vi "EminemExecute.vi"(8 "error in (no error)":errorcluster) -> (0 "error out":errorcluster)   [LabVIEW 2023]
panel:
  # "Click here to set min"
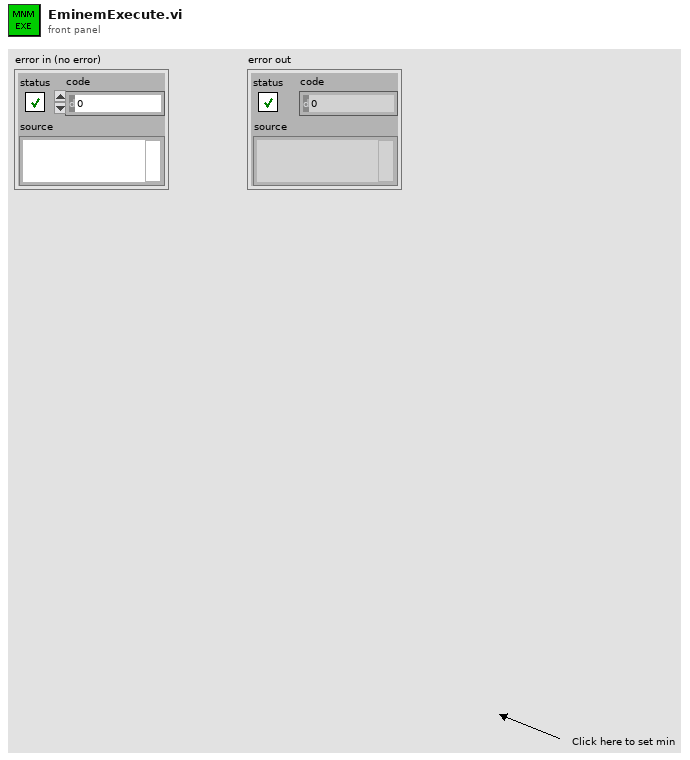
[diagram p1: front panel]
types:
  T1 = typedef "WPI_MotorControlDeviceRef.ctl" = cluster{"DeviceStatus":errorcluster, "Type":T2, "PWM":cluster{"PWM Channel":T3, "DeadBand":T4}, "CAN":cluster{"Device Number":u8, "SetOutput VI Ref":variant, "GetOutput VI Ref":variant, "Enable VI Ref":variant, "Disable VI Ref":variant, "Data":variant}, "Invert":bool, "DIO PWM":cluster{"PWM \"Enable\" Channel":T3, "DIOChannel":T5, "PWM Rate":dbl}}
  T2 = typedef "WPI_MotorControlType.ctl" = enum16{"PWM", "CAN", "DIO PWM"}
  T3 = typedef "FPGA_DIOPWMChannel.ctl" = enum8{"PWM 0", "PWM 1", "PWM 2", "PWM 3", "PWM 4", "PWM 5", "PWM 6", "PWM 7", "PWM 8", "PWM 9", "PWM MXP 0", "PWM MXP 1", "PWM MXP 2", "PWM MXP 3", "PWM MXP 4", "PWM MXP 5", "PWM MXP 6", "PWM MXP 7", "PWM MXP 8", "PWM MXP 9", "Invalid"}
  T4 = typedef "WPI_PWMDeadband.ctl" = cluster{"Name":string, "maxPositivePwm":i32, "minPositivePwm":i32, "centerPwm":i32, "maxNegativePwm":i32, "minNegativePwm":i32, "angularRange":u16}
  T5 = typedef "FPGA_DIOChannel.ctl" = enum8{"DIO 0", "DIO 1", "DIO 2", "DIO 3", "DIO 4", "DIO 5", "DIO 6", "DIO 7", "DIO 8", "DIO 9", "DIO MXP 0", "DIO MXP 1", "DIO MXP 2", "DIO MXP 3", "DIO MXP 4", "DIO MXP 5", "DIO MXP 6", "DIO MXP 7", "DIO MXP 8", "DIO MXP 9", "DIO MXP 10", "DIO MXP 11", "DIO MXP 12", "DIO MXP 13", "DIO MXP 14", "DIO MXP 15", "SPI Port CS1", "SPI Port CS2", "SPI Port CS3", "SPI Port MISO", "SPI Port MOSI", "Invalid"}
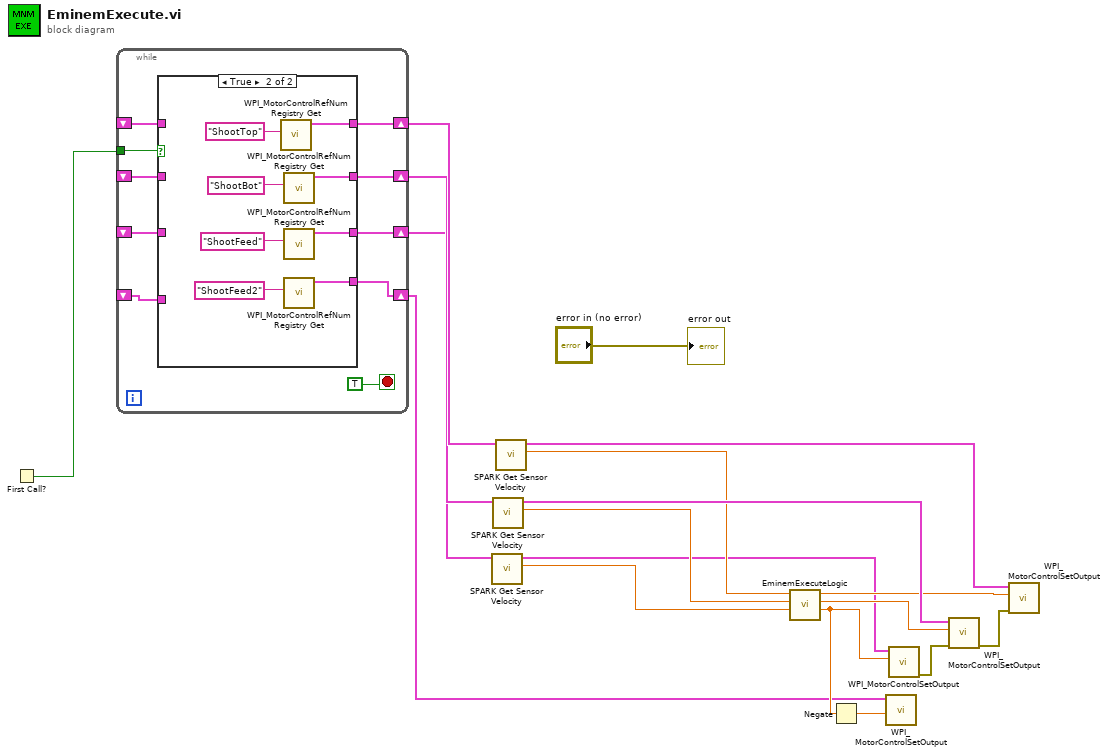
[diagram p0: block diagram]
diagram:
  n1 = First Call?() -> (First Call?: T/F=w14:bool)
  n2 = while {
    tunnel: w14 -> [w26]
    shift-right: [w28] -> w18
    shift-left: _ -> [w24]
    shift-right: [w27] -> w17
    shift-left: _ -> [w23]
    shift-right: [w22] -> w6
    shift-left: _ -> [w21]
    shift-right: [w20] -> w1
    shift-left: _ -> [w19]
    stop <- TRUE stop-if-true
    n3 = case shown="True" w26 {
      tunnel: [w32 w38] -> w28
      tunnel: [w31 w37] -> w27
      tunnel: w24 -> [w32 _]
      tunnel: w23 -> [w31 _]
      tunnel: [w30 w35] -> w22
      tunnel: w21 -> [w30 _]
      tunnel: [w29 w33] -> w20
      tunnel: w19 -> [w29 _]
      frame False {
      }
      frame True {
        n4 = call <vilib>:"WPI_MotorControlRefNum Registry Get.vi"("refnum name"="ShootTop") -> ("MotorControlDevRef"=w38:T1)  [unwired: 9 in, 1 out]
        n5 = call <vilib>:"WPI_MotorControlRefNum Registry Get.vi"("refnum name"="ShootBot") -> ("MotorControlDevRef"=w37:T1)  [unwired: 9 in, 1 out]
        n6 = call <vilib>:"WPI_MotorControlRefNum Registry Get.vi"("refnum name"="ShootFeed") -> ("MotorControlDevRef"=w35:T1)  [unwired: 9 in, 1 out]
        n7 = call <vilib>:"WPI_MotorControlRefNum Registry Get.vi"("refnum name"="ShootFeed2") -> ("MotorControlDevRef"=w33:T1)  [unwired: 9 in, 1 out]
      }
    }
  }
  n8 = call <vilib>:"SPARK Get Sensor Velocity.vi"("MotorControlDevRef in"=w6) -> ("Sensor Velocity"=w4:dbl, "MotorControlDevRef out"=w5:T1)  [unwired: 7 in, 2 out]
  n9 = call <vilib>:"SPARK Get Sensor Velocity.vi"("MotorControlDevRef in"=w17) -> ("Sensor Velocity"=w10:dbl, "MotorControlDevRef out"=w16:T1)  [unwired: 7 in, 2 out]
  n10 = call <vilib>:"SPARK Get Sensor Velocity.vi"("MotorControlDevRef in"=w18) -> ("Sensor Velocity"=w11:dbl, "MotorControlDevRef out"=w7:T1)  [unwired: 7 in, 2 out]
  n11 = call "EminemExecuteLogic.vi"("Feed_Vel_RPM"=w4, "Shooter_Bottom_Vel_RPM"=w10, "Shooter_Top_Vel_RPM"=w11) -> ("Shooter_Feed_Motor_Out"=w2:dbl, "Shooter_Bottom_Motor_Out"=w8:dbl, "Shooter_Top_Motor_Out"=w9:dbl)  [unwired: 5 in, 1 out]
  n12 = Negate(x=w2) -> (-x=w3:dbl)
  n13 = call <vilib>:"WPI_MotorControlSetOutput.vi"("Output"=w3, "MotorControlDevRef"=w1) -> ()  [unwired: 7 in, 3 out]
  n14 = call <vilib>:"WPI_MotorControlSetOutput.vi"("Output"=w2, "MotorControlDevRef"=w5) -> ("error out"=w13:errorcluster)  [unwired: 7 in, 2 out]
  n15 = call <vilib>:"WPI_MotorControlSetOutput.vi"("error in (no error)"=w13, "Output"=w8, "MotorControlDevRef"=w16) -> ("error out"=w12:errorcluster)  [unwired: 6 in, 2 out]
  n16 = call <vilib>:"WPI_MotorControlSetOutput.vi"("error in (no error)"=w12, "Output"=w9, "MotorControlDevRef"=w7) -> ()  [unwired: 6 in, 3 out]
  "error out" <- "error in (no error)"
